vi "lsl append child.vi"(8 "error in (no error)":errorcluster, 10 "name":string, 11 "xml_ptr":u64) -> (0 "error out":errorcluster, 2 "function return":u32, 3 "xml_ptr 2":u64)   [LabVIEW 2016, in "Lab Streaming Layer.lvlib"]
doc: "extern LIBLSL_C_API lsl_xml_ptr lsl_append_child(lsl_xml_ptr e, const char *name);"
uses:
  Lab Streaming Layer.lvlib
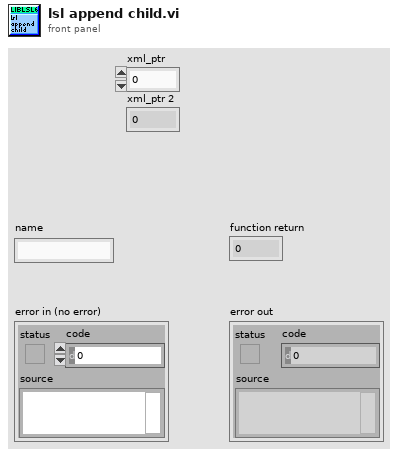
[diagram p1: front panel]
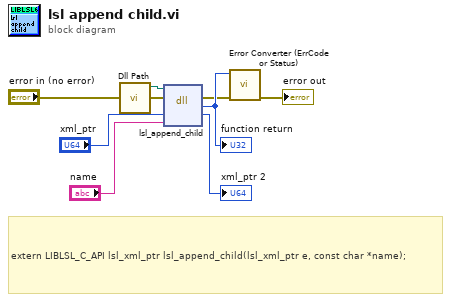
[diagram p0: block diagram]
diagram:
  # "extern LIBLSL_C_API lsl_xml_ptr lsl_append_child(lsl_xml_ptr e, const char *name);"
  n1 = call "Dll Path.vi"() -> ("Dll path"=w1:path)  [unwired: 11 in]
  n2 = dll-call lib="E:/LabStreamingLayer/liblsl-LabVIEW-master/liblsl-LabVIEW-master/lsl.dll" fn="lsl_append_child"(path in=w1, error in="error in (no error)", "xml_ptr"="xml_ptr", "name"="name") -> (error out=w5:errorcluster, "return type"=w8:u32, "xml_ptr"=→"xml_ptr 2":u64)  [unwired: 2 in, 1 out]
  "function return" <- w8
  n3 = call "Error Converter (ErrCode or Status).vi"("error in (no error)"=w5, "error code"=w8) -> ("error out"=→"error out":errorcluster)  [unwired: 9 in]
